vi "ToTable.vi"(8 "error in":errorcluster, 9 "Table Index (0)":i32, 10 "variant":variant, 11 "SystemLin Tag Module editor node in":refnum<class "SystemLink File editor node.lvclass">) -> (0 "error out":errorcluster, 1 "row headers":string[](array[string]), 2 "table":string[][](array[string]), 3 "SystemLin Tag Module editor node out":refnum<class "SystemLink File editor node.lvclass">)   [LabVIEW 2015, in "SystemLink File editor node.lvclass"]
doc: "Generates the strings needed to display on a table based on the information found in the engine and module configuration classes."
uses:
  SystemLink File editor node.lvclass
  module/configuration/SystemLink File configuration.lvclass
  <vilib>/NI/Module Execution Interface/Engine Configuration/engine configuration.lvclass
  <vilib>/NI/Configuration Framework/serializable configuration/NISE_CEF_serializable configuration.lvclass/NISE_CEF_serializable configuration.ctl
  <vilib>/NI/Tag Bus/tag/tag descriptor.lvclass/tag descriptor.ctl
  <vilib>/Utility/LVClass/Get LV Class Name.vi
  <vilib>/NI/Configuration Framework/error generator/NISE_error generator.vi
  <vilib>/NI/Tag Bus/tag/default value polymorphs/read default value Boolean.vi
  <vilib>/NI/Tag Bus Module Framework/channel/TBM channel.lvclass
  <vilib>/NI/Tag Bus/tag/tag descriptor.lvclass
  <vilib>/NI/Configuration Framework/serializable configuration/NISE_CEF_serializable configuration.lvclass
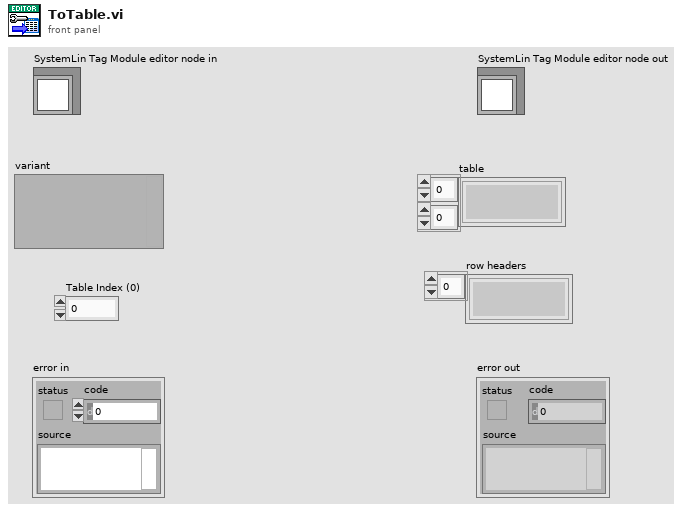
[diagram p1: front panel]
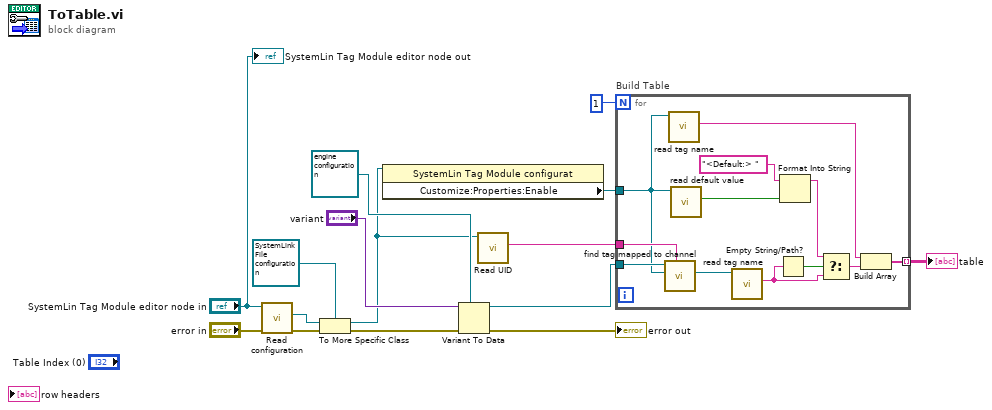
[diagram p0: block diagram]
diagram:
  n1 = call-dynamic "Read configuration.vi"("error in"="error in", "SystemLin Tag Module editor node in"="SystemLin Tag Module editor node in") -> ("error out"=w15:errorcluster, "configuration"=w6:refnum<class "NISE_CEF_serializable configuration.lvclass">)  [unwired: 7 in, 1 out]
  n2 = To More Specific Class(target class=refnum<class "SystemLink File configuration.lvclass"> refnum ("tag bus configurable plugin module configuration"), reference=w6, error in=w15) -> (specific class reference=w5:refnum<class "SystemLink File configuration.lvclass">, error out=w3:errorcluster)
  n3 = property class="SystemLin Tag Module configurat"(reference=w5) -> ("Customize:Properties:Enable"=w12:refnum<class "TBM channel.lvclass">)  [unwired: 1 in, 2 out]
  n4 = Variant To Data(error in=w3, type=refnum<class "engine configuration.lvclass"> refnum ("engine configuration"), Variant="variant") -> (data=w9:refnum<class "engine configuration.lvclass">, error out=→"error out":errorcluster)
  n5 = call <vilib>:"Read UID.vi"("configuration in"=w5) -> ("instance id"=w4:string)  [unwired: 8 in, 2 out]
  n6 = for "Build Table" {
    N: 1 -> [_]
    tunnel: w12 -> [w22]
    tunnel: w9 -> [w26]
    tunnel: [w24] -> w7 mode=indexing
    tunnel: w4 -> [w23]
    n7 = call <vilib>:"find tag mapped to channel.vi"("owner"=w23, "channel"=w22, "engine configuration in"=w26) -> ("tag"=w25:refnum<class "tag descriptor.lvclass">)  [unwired: 6 in, 2 out]
    n8 = call <vilib>:"read tag name.vi"("system tag in"=w22) -> ("name"=w27:string)  [unwired: 8 in, 2 out]
    n9 = call-poly <vilib>:"read default value.vi"("system tag in"=w22) -> ("default value"=w21:bool)  [unwired: 7 in, 3 out]
    n10 = call <vilib>:"read tag name.vi"("system tag in"=w25) -> ("name"=w17:string)  [unwired: 8 in, 2 out]
    n11 = Empty String/Path?(string/path=w17) -> (empty?=w19:bool)
    n12 = Format Into String(initial string="<Default:> ", w21) -> (resulting string=w18:string)  [unwired: 2 in, 1 out]
    n13 = Select(t=w18, s=w19, f=w17) -> (s? t:f=w16:string)
    n14 = Build Array(w27, w16) -> (w24:string[])
  }
  "table" <- w7
  "SystemLin Tag Module editor node out" <- "SystemLin Tag Module editor node in"
